vi "crio_FPGA_LAC.vi"() -> ()   [LabVIEW 2019]
uses:
  <vilib>/rvi/Emulation/niFpgaSctlEmulationGetInTimedLoop.vi
  <vilib>/rvi/Emulation/niFpgaProcessEmulError.vi
  <vilib>/rvi/eio/common/nirviEmuTemplateMethod_errors.vi
  <vilib>/rvi/Emulation/niFpgaGetClockAttributes.vi
  <vilib>/rvi/Emulation/niFpgaEmulationReportErrorSimple.vi
  <vilib>/rvi/Emulation/niFpgaCriticalErrorInLSC.vi
  <vilib>/eio/EIOMethodNode/EIOMethodNode.xnode
  <vilib>/eio/EIONode/EIONode.xnode
panel:
  in  "LAC Lock":bool
  in  "Debug: ConnectorA/DIO15":bool
  in  "Debug: ConnectorA/DIO14":bool
  in  "Encoder Debug":bool
  in  "Loop Timer DAQ":u32=1 caption="Loop Time(uSec)"
  in  "Position Reset":bool
  out "Position (Counts)":i64
  out "B":bool
  out "A":bool
  out "B'":bool
  out "A'":bool
  in  "Velocity Interval (uSec)":u32=1000
  out "Acceleration (Counts/Interval)":i32
  out "Velocity (Counts/Interval)":i32
  in  "stop":bool
  in  "Servo wait time":u32(slide)=828 scale=1000.0..2000.0
  in  "Count(uSec)":u32=2000
  # "1000, fully retract\n2000, fully extend\nbetween, inner PD control"
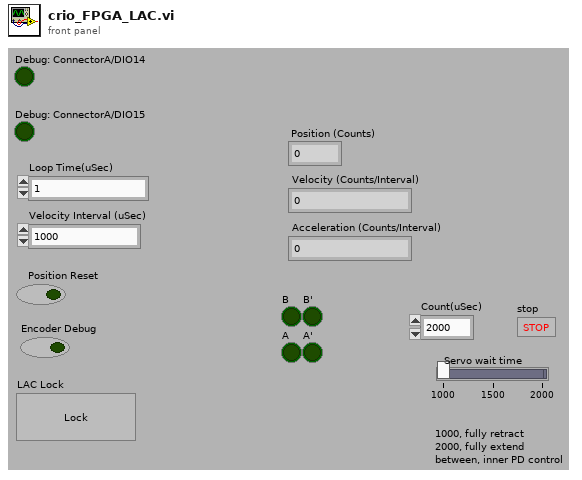
[diagram p1: front panel]
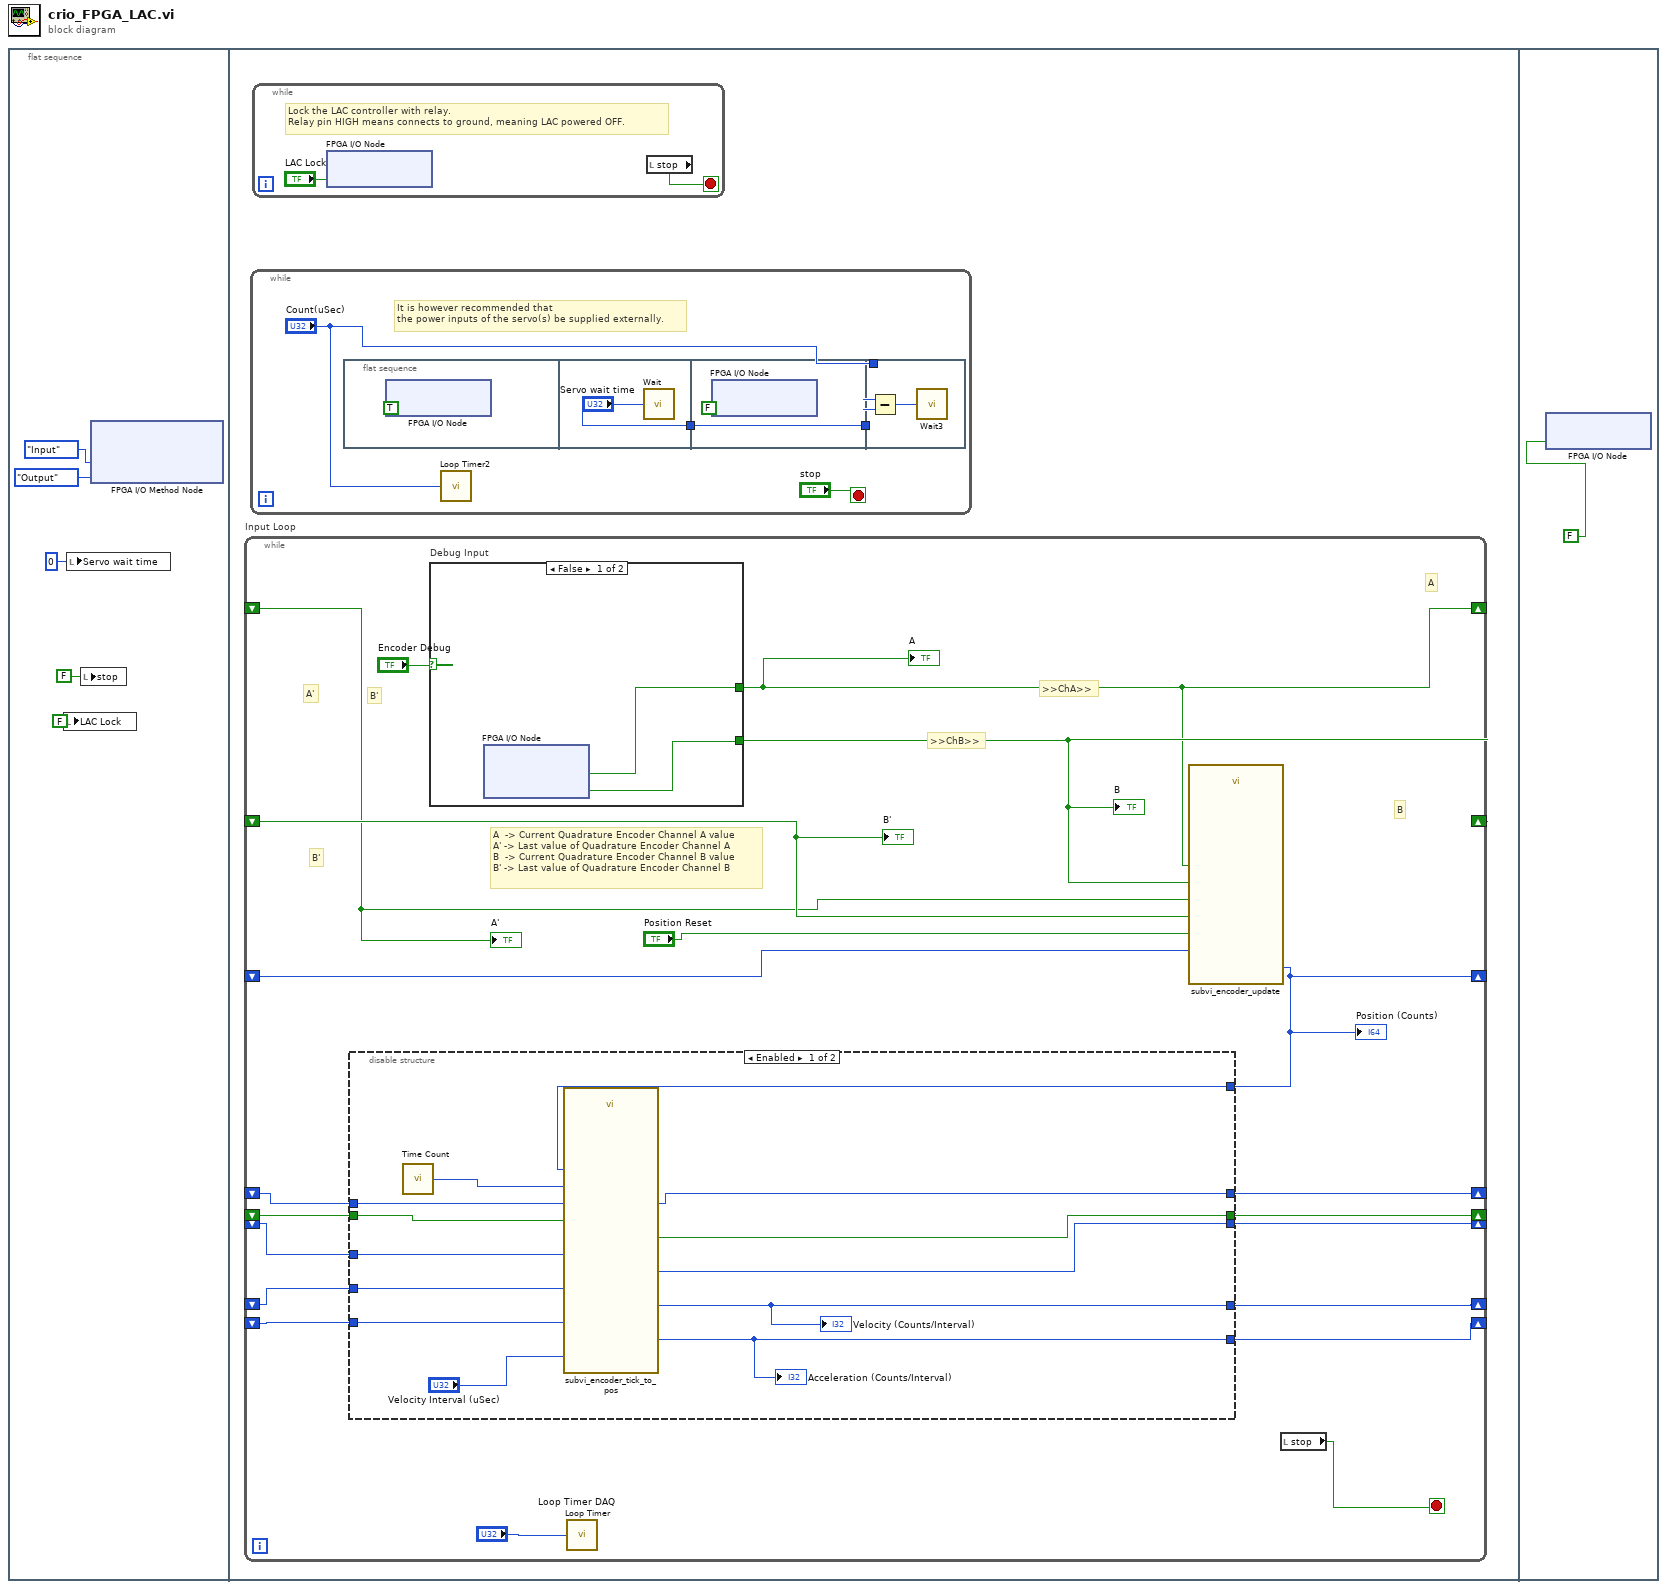
[diagram p0: block diagram]
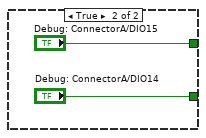
[diagram p3: hidden frame]
diagram:
  n1 = flat-sequence {
    frame #0 {
      n2 = local write "LAC Lock"(FALSE ("Lock")) -> ()
      n3 = local write "Servo wait time"(u32 0 ("Servo wait time")) -> ()
      n4 = local write "stop"(FALSE ("stop")) -> ()
      n5 = xnode "FPGA I/O Method Node"("DIO 7:4"=enum8{"No Change", "Input", "Output"}."Input", "DIO 3:0"=enum8{"No Change", "Input", "Output"}."Output") -> ()  [unwired: 1 in, 1 out]
    }
    frame #1 {
      n6 = while "Input Loop" {
        shift-right: [w21] -> _
        shift-left: _ -> [w24]
        shift-right: [w20] -> _
        shift-left: _ -> [w23]
        shift-right: [w16] -> _
        shift-left: _ -> [w22]
        shift-right: [w9] -> _
        shift-left: _ -> [w19]
        shift-right: [w10] -> _
        shift-left: _ -> [w18]
        shift-right: [w17] -> _
        shift-left: _ -> [w15]
        shift-right: [w14] -> _
        shift-left: _ -> [w13]
        shift-right: [w12] -> _
        shift-left: _ -> [w11]
        stop <- w8 stop-if-true
        # "B'"
        # ">>ChB>>"
        # ">>ChA>>"
        # "A'"
        # "A  -> Current Quadrature Encoder Channel A value\nA' -> Last value of Quadrature Encoder Channel A\nB  -> Current Quadrature Encoder Channel B value\nB' -> Last value of Quadrature Encoder Channel B"
        # "B'"
        # "B"
        # "A"
        n7 = case "Debug Input" shown="False" "Encoder Debug" {
          tunnel: [w42 "Debug: ConnectorA/DIO15"] -> w20
          tunnel: [w41 "Debug: ConnectorA/DIO14"] -> w21
          frame False {
            n8 = xnode "FPGA I/O Node"() -> ("Mod2/DIO2"=w42:bool, "Mod2/DIO3"=w41:bool)  [unwired: 2 in, 2 out]
          }
          frame True {
          }
        }
        "B" <- w21
        "A" <- w20
        n9 = call "Loop Timer"("Count(uSec)"="Loop Timer DAQ") -> ()  [unwired: 1 out]
        n10 = call "subvi_encoder_update.vi"("Position Reset"="Position Reset", "Tick'"=w22, "A"=w20, "B'"=w24, "A'"=w23, "B"=w21) -> ("Tick"=w16:i32)  [unwired: 5 in]
        "Position (Counts)" <- w16
        n11 = disable-structure shown="Enabled" {
          disable-tunnel: w19 -> [w39 _]
          disable-tunnel: w18 -> [w38 _]
          disable-tunnel: [w37 _] -> w17
          disable-tunnel: w16 -> [w36 _]
          disable-tunnel: w15 -> [w35 _]
          disable-tunnel: [w34 _] -> w14
          disable-tunnel: w13 -> [w33 _]
          disable-tunnel: [w32 _] -> w12
          disable-tunnel: w11 -> [w31 _]
          disable-tunnel: [w29 _] -> w10
          disable-tunnel: [w28 _] -> w9
          frame Enabled {
            n12 = call "Time Count"() -> ("Tick Count(uSec)"=w30:u32)
            n13 = call "subvi_encoder_tick_to_pos.vi"("Velocity Interval (uSec)"="Velocity Interval (uSec)", "Raw Tick"=w36, "Waited?'"=w33, "Tick Count(uSec)'"=w31, "p'"=w35, "Time Count"=w30, "a'"=w38, "v'"=w39) -> ("Waited?"=w34:bool, "Tick Count(uSec)"=w32:u32, "p"=w37:i32, "a"=w29:i32, "v"=w28:i32)  [unwired: 3 in]
            "Acceleration (Counts/Interval)" <- w29
            "Velocity (Counts/Interval)" <- w28
          }
          frame Disabled {
          }
        }
        n14 = local read "stop"() -> (w8:bool)
        "B'" <- w24
        "A'" <- w23
      }
      n15 = while {
        stop <- "stop" stop-if-true
        # "It is however recommended that\nthe power inputs of the servo(s) be supplied externally."
        n16 = flat-sequence {
          tunnel: ["Servo wait time"] -> w46
          tunnel: [w51] -> w47
          tunnel: w46 -> [w51]
          tunnel: "Count(uSec)" -> [w55]
          tunnel: w47 -> [w54]
          frame #0 {
            n17 = xnode "FPGA I/O Node"("Mod8/DIO5"=TRUE) -> ()  [unwired: 1 in, 1 out]
          }
          frame #1 {
            n18 = call "Wait"("Count(uSec)"="Servo wait time") -> ()  [unwired: 1 out]
          }
          frame #2 {
            n19 = xnode "FPGA I/O Node"("Mod8/DIO5"=FALSE) -> ()  [unwired: 1 in, 1 out]
          }
          frame #3 {
            n20 = Subtract(x=w55, y=w54) -> (x-y=w53:u32)
            n21 = call "Wait3"("Count(uSec)"=w53) -> ()  [unwired: 1 out]
          }
        }
        n22 = call "Loop Timer2"("Count(uSec)"="Count(uSec)") -> ()  [unwired: 1 out]
      }
      n23 = while {
        stop <- w7 stop-if-true
        # "Lock the LAC controller with relay.\nRelay pin HIGH means connects to ground, meaning LAC powered OFF."
        n24 = xnode "FPGA I/O Node"("Mod8/DIO6"="LAC Lock") -> ()  [unwired: 1 in, 1 out]
        n25 = local read "stop"() -> (w7:bool)
      }
    }
    frame #2 {
      n26 = xnode "FPGA I/O Node"("Mod8/DIO5"=FALSE) -> ()  [unwired: 1 in, 1 out]
    }
  }
